vi "过滤筛选流程.vi"(11 "字符串":string) -> (3 "匹配后偏移量":i32)   [LabVIEW 2016, in "斯坦道总氮V2.lvlib"]
uses:
  <vilib>/regexp/Match Regular Expression.xnode
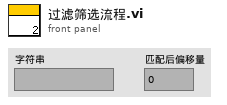
[diagram p1: front panel]
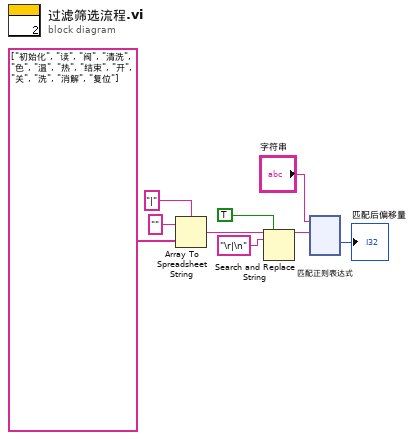
[diagram p0: block diagram]
diagram:
  n1 = Array To Spreadsheet String(delimiter (Tab)="|" ("分隔符(Tab)"), array=string[] ["初始化", "读", "阀", "清洗", "色", "温", "热", "结束", "开", "关", "洗", "消解", "复位"], 3:"" ("格式字符串")) -> (spreadsheet string=w5:string)
  n2 = Search and Replace String(replace all?=TRUE ("替换全部？(F)"), input string=w5, search string="\r|\n" ("搜索字符串")) -> (result string=w4:string)  [unwired: 5 in, 3 out]
  n3 = xnode "匹配正则表达式"("输入字符串"="字符串", "正则表达式"=w4) -> ("匹配后偏移量"=→"匹配后偏移量":i32)  [unwired: 4 in, 4 out]
